vi "Stop.vi"(6 "Busy":refnum<vi>, 8 "error in (no error)":errorcluster, 11 "Motor in":refnum<class "Motor.lvclass">) -> (0 "error out":errorcluster, 2 "String":string, 3 "Motor out":refnum<class "Motor.lvclass">)   [LabVIEW 2018, in "Motor.lvclass"]
uses:
  Motor.lvclass
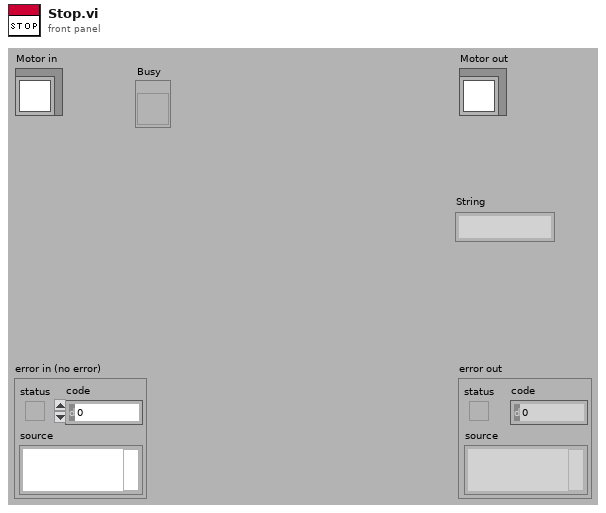
[diagram p1: front panel]
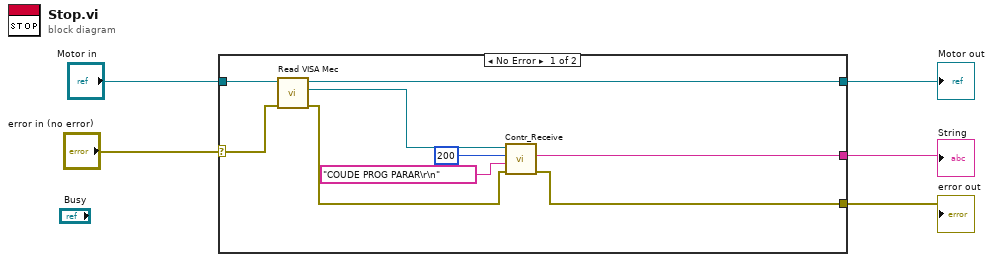
[diagram p0: block diagram]
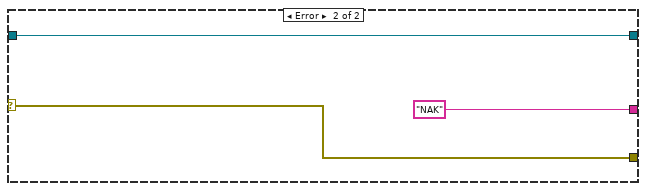
[diagram p2: hidden frame]
diagram:
  n1 = case shown="No Error" "error in (no error)" {
    selector: "error in (no error)" -> [w8 w17]
    tunnel: "Motor in" -> [w10 w16]
    tunnel: [w9 w16] -> w3
    tunnel: [w11 w17] -> w2
    tunnel: [w6 "NAK" ("Response from SIFS")] -> w1
    frame No Error {
      n2 = call-dynamic "Read VISA Mec.vi"("error in (no error)"=w8, "Controlador in"=w10) -> ("error out"=w7:errorcluster, "VISA Mec"=w13:refnum<visa-resource-name>, "Controlador out"=w9:refnum<class "Motor.lvclass">)  [unwired: 7 in]
      n3 = call "Contr_Receive.vi"("error in"=w7, "Command to SIFS"="COUDE PROG PARAR\r\n", "wait after tx"=u32 200, "VISA resource name"=w13) -> ("error out"=w11:errorcluster, "Response from SIFS"=w6:string)  [unwired: 2 out]
    }
    frame Error {
    }
  }
  "error out" <- w2
  "Motor out" <- w3
  "String" <- w1
